vi "Disabled - Const Output to Cluster (SubVI).vi"(7 "Constants Numeric Array":dbl[](array[numeric]), 11 "Constant Input Cluster":T1) -> (3 "Constant Cluster":T1)   [LabVIEW 2018]
uses:
  Disabled - Constant Cluster Typedef.ctl
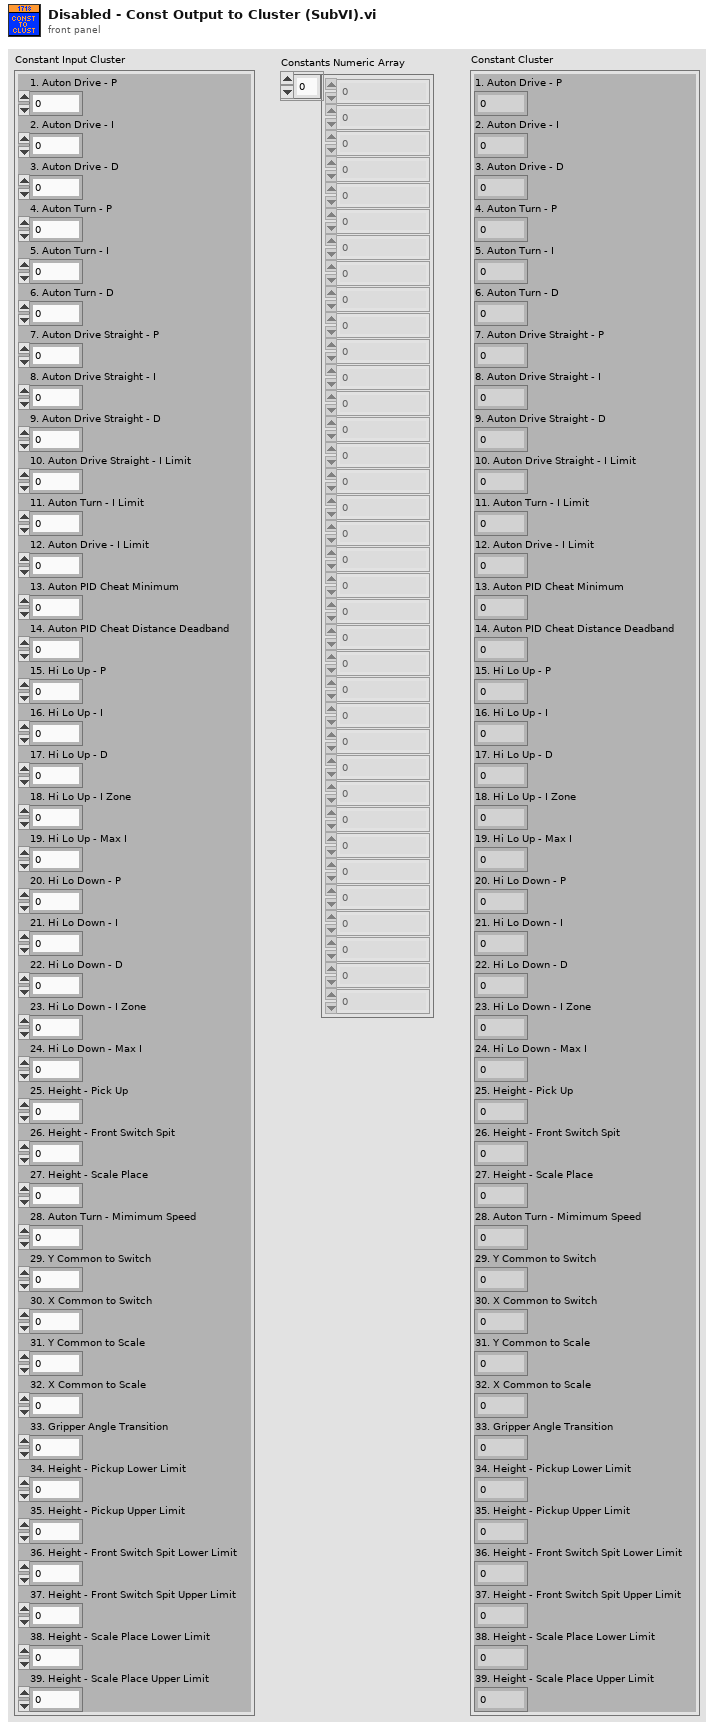
[diagram p1: front panel]
types:
  T1 = typedef "Disabled - Constant Cluster Typedef.ctl" = cluster{"1. Auton Drive - P":dbl, "2. Auton Drive - I":dbl, "3. Auton Drive - D":dbl, "4. Auton Turn - P":dbl, "5. Auton Turn - I":dbl, "6. Auton Turn - D":dbl, "7. Auton Drive Straight - P":dbl, "8. Auton Drive Straight - I":dbl, "9. Auton Drive Straight - D":dbl, "10. Auton Drive Straight - I Limit":dbl, "11. Auton Turn - I Limit":dbl, "12. Auton Drive - I Limit":dbl, "13. Auton PID Cheat Minimum":dbl, "14. Auton PID Cheat Distance Deadband":dbl, "15. Hi Lo Up - P":dbl, "16. Hi Lo Up - I":dbl, "17. Hi Lo Up - D":dbl, "18. Hi Lo Up - I Zone":dbl, "19. Hi Lo Up - Max I":dbl, "20. Hi Lo Down - P":dbl, "21. Hi Lo Down - I":dbl, "22. Hi Lo Down - D":dbl, "23. Hi Lo Down - I Zone":dbl, "24. Hi Lo Down - Max I":dbl, "25. Height - Pick Up":dbl, "26. Height - Front Switch Spit":dbl, "27. Height - Scale Place":dbl, "28. Auton Turn - Mimimum Speed":dbl, "29. Y Common to Switch":dbl, "30. X Common to Switch":dbl, "31. Y Common to Scale":dbl, "32. X Common to Scale":dbl, "33. Gripper Angle Transition":dbl, "34. Height - Pickup Lower Limit":dbl, "35. Height - Pickup Upper Limit":dbl, "36. Height - Front Switch Spit Lower Limit":dbl, "37. Height - Front Switch Spit Upper Limit":dbl, "38. Height - Scale Place Lower Limit":dbl, "39. Height - Scale Place Upper Limit":dbl}
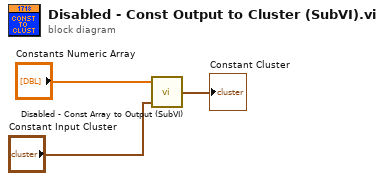
[diagram p0: block diagram]
diagram:
  n1 = call "Disabled - Const Array to Output (SubVI).vi"("Constant cluster"="Constant Input Cluster", "Constants Numeric Array"="Constants Numeric Array") -> ("Constant cluster output"=→"Constant Cluster":T1)  [unwired: 2 in]
